vi "KM101_ReadPosition.vi"(9 "Channel":i32, 10 "reference in":refnum<k7>) -> (1 "Steps":i32, 2 "reference out":refnum<k7>)   [LabVIEW 2018, in "KIM101lib.lvlib"]
uses:
  KIM101lib.lvlib
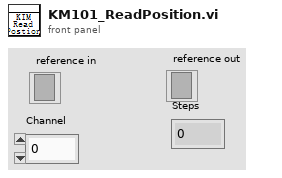
[diagram p1: front panel]
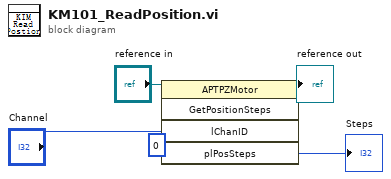
[diagram p0: block diagram]
diagram:
  n1 = invoke class="APTPZMotor" method="GetPositionSteps"(reference="reference in", "lChanID"="Channel", "plPosSteps"=0) -> (reference out=→"reference out":refnum<k7>, "plPosSteps"=→"Steps":i32)  [unwired: 2 in, 3 out]
